vi "LevMar - TestSuite.vi"() -> ()   [LabVIEW 2009]
uses:
  <vilib>/Analysis/NI_AALBase.lvlib
panel:
  out "Reduced Chi2":dbl(graph)=0.8280414251118929
  out "Graphe XY":T1(graph)=[{"Ramp Pattern"=[-1.0, -0.9797979797979798, -0.9595959595959596, -0.9393939393939393, -0.9191919191919191, -0.8989898989898989, -0.8787878787878787, -0.8585858585858585, -0.8383838383838382, -0.818181818181818, -0.7979797979797978, -0.7777777777777776, -0.7575757575757573, -0.7373737373737371, -0.7171717171717169, -0.6969696969696967, -0.6767676767676765, -0.6565656565656562, -0.636363636363636, -0.6161616161616158, -0.5959595959595956, -0.5757575757575754, -0.5555555555555551, -0.5353535353535349, -0.5151515151515147, -0.4949494949494945, -0.47474747474747425, -0.45454545454545403, -0.4343434343434338, -0.4141414141414136, -0.39393939393939337, -0.37373737373737315, -0.3535353535353529, -0.3333333333333327, -0.3131313131313125, -0.29292929292929226, -0.27272727272727204, -0.2525252525252518, -0.23232323232323163, -0.21212121212121143, -0.19191919191919124, -0.17171717171717105, -0.15151515151515085, -0.13131313131313066, -0.11111111111111045, -0.09090909090909025, -0.07070707070707004, -0.05050505050504983, -0.030303030303029627, -0.010101010101009424, 0.01010101010101078, 0.030303030303030984, 0.05050505050505119, 0.0707070707070714, 0.0909090909090916, 0.11111111111111181, 0.13131313131313202, 0.1515151515151522, 0.1717171717171724, 0.1919191919191926, 0.2121212121212128, 0.232323232323233, 0.2525252525252532, 0.27272727272727343, 0.29292929292929365, 0.31313131313131387, 0.3333333333333341, 0.3535353535353543, 0.37373737373737453, 0.39393939393939476, 0.414141414141415, 0.4343434343434352, 0.4545454545454554, 0.47474747474747564, 0.49494949494949586, 0.515151515151516, 0.5353535353535362, 0.5555555555555565, 0.5757575757575767, 0.5959595959595969, 0.6161616161616171, 0.6363636363636374, 0.6565656565656576, 0.6767676767676778, 0.696969696969698, 0.7171717171717182, 0.7373737373737385, 0.7575757575757587, 0.7777777777777789, 0.7979797979797991, 0.8181818181818193, 0.8383838383838396, 0.8585858585858598, 0.87878787878788, 0.8989898989899002, 0.9191919191919204, 0.9393939393939407, 0.9595959595959609, 0.9797979797979811, 1.0000000000000013], "Best Fit"=[-0.0016898079029579738, -0.010518321765782213, -0.01737091840455096, -0.022296729825936557, -0.025344888036609614, -0.026564525043242138, -0.026004772852505242, -0.023714763471070988, -0.019743628905610155, -0.01414050116279486, -0.006954512249295941, 0.0017652058282146, 0.011969521063065702, 0.023609301448585474, 0.03663541497810291, 0.05099872964494598, 0.06665011344244379, 0.08354043436392442, 0.10162056040271661, 0.12084135955214889, 0.14115369980554973, 0.16250844915624768, 0.18485647559757126, 0.20814864712284895, 0.2323358317254094, 0.257368897398581, 0.2831987121356923, 0.3097761439300718, 0.3370520607750481, 0.36497733066394983, 0.3935028215901053, 0.4225794015468432, 0.452157938527492, 0.4821893005253801, 0.5126243555338362, 0.5434139715461888, 0.5745090165557664, 0.6058603585558975, 0.6374188655399105, 0.6691354055011342, 0.7009608464328968, 0.7328460563285272, 0.7647419031813537, 0.7965992549847049, 0.8283689797319093, 0.8600019454162954, 0.8914490200311918, 0.9226610715699269, 0.9535889680258294, 0.9841835773922277, 1.0143957676624504, 1.0441764068298258, 1.0734763628876829, 1.1022465038293496, 1.130437697648155, 1.1580008123374275, 1.1848867158904952, 1.211046276300687, 1.2364303615613315, 1.260989839665757, 1.2846755786072923, 1.3074384463792654, 1.3292293109750055, 1.3499990403878406, 1.3696985026110995, 1.3882785656381107, 1.4056900974622026, 1.421883966076704, 1.436811039474943, 1.4504221856502484, 1.4626682725959488, 1.4735001683053726, 1.4828687407718482, 1.4907248579887042, 1.4970193879492693, 1.5017031986468719, 1.5047271580748405, 1.5060421342265038, 1.50559899509519, 1.5033486086742278, 1.499241842956946, 1.4932295659366728, 1.4852626456067366, 1.4752919499604662, 1.4632683469911902, 1.4491427046922367, 1.4328658910569347, 1.4143887740786125, 1.3936622217505985, 1.3706371020662216, 1.34526428301881, 1.317494632601692, 1.287279018808197, 1.254568309631653, 1.219313373065388, 1.1814650771027315, 1.1409742897370114, 1.0977918789615562, 1.051868712769695, 1.0031556591547555]}, {"Ramp Pattern"=[-1.0, -0.9797979797979798, -0.9595959595959596, -0.9393939393939393, -0.9191919191919191, -0.8989898989898989, -0.8787878787878787, -0.8585858585858585, -0.8383838383838382, -0.818181818181818, -0.7979797979797978, -0.7777777777777776, -0.7575757575757573, -0.7373737373737371, -0.7171717171717169, -0.6969696969696967, -0.6767676767676765, -0.6565656565656562, -0.636363636363636, -0.6161616161616158, -0.5959595959595956, -0.5757575757575754, -0.5555555555555551, -0.5353535353535349, -0.5151515151515147, -0.4949494949494945, -0.47474747474747425, -0.45454545454545403, -0.4343434343434338, -0.4141414141414136, -0.39393939393939337, -0.37373737373737315, -0.3535353535353529, -0.3333333333333327, -0.3131313131313125, -0.29292929292929226, -0.27272727272727204, -0.2525252525252518, -0.23232323232323163, -0.21212121212121143, -0.19191919191919124, -0.17171717171717105, -0.15151515151515085, -0.13131313131313066, -0.11111111111111045, -0.09090909090909025, -0.07070707070707004, -0.05050505050504983, -0.030303030303029627, -0.010101010101009424, 0.01010101010101078, 0.030303030303030984, 0.05050505050505119, 0.0707070707070714, 0.0909090909090916, 0.11111111111111181, 0.13131313131313202, 0.1515151515151522, 0.1717171717171724, 0.1919191919191926, 0.2121212121212128, 0.232323232323233, 0.2525252525252532, 0.27272727272727343, 0.29292929292929365, 0.31313131313131387, 0.3333333333333341, 0.3535353535353543, 0.37373737373737453, 0.39393939393939476, 0.414141414141415, 0.4343434343434352, 0.4545454545454554, 0.47474747474747564, 0.49494949494949586, 0.515151515151516, 0.5353535353535362, 0.5555555555555565, 0.5757575757575767, 0.5959595959595969, 0.6161616161616171, 0.6363636363636374, 0.6565656565656576, 0.6767676767676778, 0.696969696969698, 0.7171717171717182, 0.7373737373737385, 0.7575757575757587, 0.7777777777777789, 0.7979797979797991, 0.8181818181818193, 0.8383838383838396, 0.8585858585858598, 0.87878787878788, 0.8989898989899002, 0.9191919191919204, 0.9393939393939407, 0.9595959595959609, 0.9797979797979811, 1.0000000000000013], "Best Fit"=[0.0068763694567000105, -0.013757383340708685, -0.0272231962940259, -0.021606159820455873, -0.029952272522872393, -0.02794214384950997, -0.041467239064541625, -0.021168592799294707, -0.02474381389419588, 0.00267259751288184, -0.0010875078317083104, 0.006935196863699051, 0.02371014280289723, 0.024350215775652204, 0.035589174010403776, 0.06445808144428938, 0.07683458790373367, 0.08183637710296356, 0.09127531613198694, 0.12416245979065038, 0.1383160631505338, 0.15870717638953083, 0.18896831456394578, 0.19214243850283919, 0.2459083674187535, 0.2547635484506904, 0.2705573482370152, 0.3140520910654134, 0.34446844589872927, 0.3503785326623043, 0.3774173461312958, 0.41026332139838784, 0.4573052751472374, 0.4806701569394728, 0.49319035392745986, 0.5473355214834735, 0.5814913095186334, 0.6003332277431696, 0.6359363831011836, 0.6847120296522752, 0.6979898441718131, 0.7318336707796799, 0.7678382522048454, 0.806270615423049, 0.8227181691173335, 0.8648107494305103, 0.885698597958113, 0.9444874055653282, 0.9678084783900404, 0.9870660398026526, 1.0117064267265494, 1.02885879678619, 1.0776699526365756, 1.103032050385832, 1.1240294227010545, 1.1579427056971643, 1.198048582057967, 1.2004426344631474, 1.239306308869129, 1.2679423130993166, 1.2862664199719294, 1.3089566783906899, 1.3296856943335784, 1.3477340839541145, 1.3501324109053527, 1.4024117914777718, 1.3990612113567793, 1.4177994589161165, 1.4536408827705687, 1.4428389277741696, 1.459603383882423, 1.4790749393406786, 1.4688628194274158, 1.4779910036411437, 1.4886019053135138, 1.5192068140825437, 1.5056057062591697, 1.5112645805524276, 1.5059178390597947, 1.5131001873938164, 1.5000642610260897, 1.5006317922343897, 1.49826796404352, 1.4847408656101546, 1.4584376620416672, 1.4451782789969199, 1.4212354477953029, 1.3992929656483506, 1.3888595982023753, 1.358099138788165, 1.3392365798120078, 1.3158770982609125, 1.2900307263125528, 1.2521637211322305, 1.2347895389871848, 1.1717961456379768, 1.1433511019909486, 1.1082589909107459, 1.0540896400505515, 1.0037091247691126]}]
  in  "standard deviation":dbl=0.009999999999999997 caption="écart-type" format="%.6f"
  out "Best Fit Coefficients":dbl[](array[numeric])=[0.9993405456647769, 1.4956047531397814, -0.49860762003887654, -0.993182019610923] caption="Coefficients d'ajustement optimaux" format="%_6f"
  in  "A":dbl[](array[numeric])=[1.0, 1.5, -0.5, -1.0]
  in  "samples":i32=100 caption="échantillons"
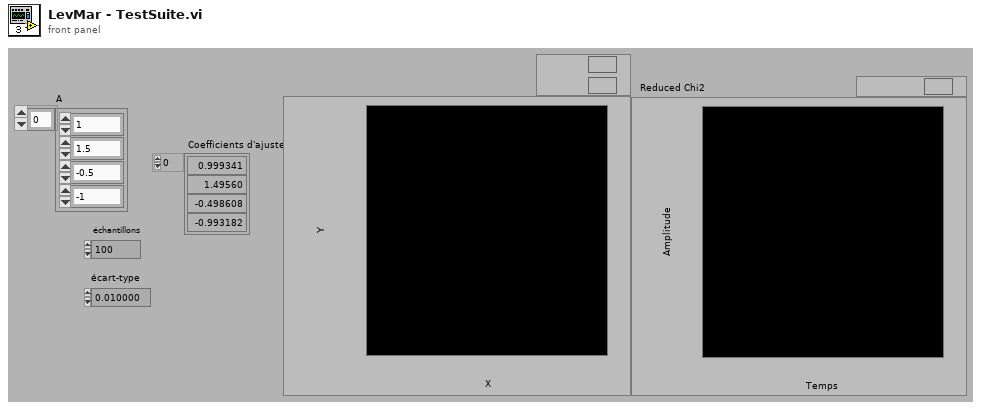
[diagram p1: front panel]
types:
  T1 = cluster{"Ramp Pattern":dbl[], "Best Fit":dbl[]}[]
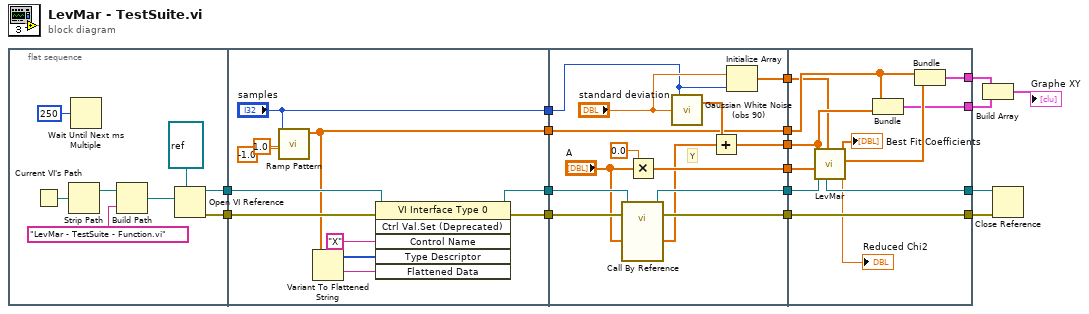
[diagram p0: block diagram]
diagram:
  n1 = flat-sequence {
    tunnel: [w20] -> w17
    tunnel: [w19] -> w16
    tunnel: w16 -> [w34]
    tunnel: w17 -> [w35]
    tunnel: [w35] -> w15
    tunnel: [w33] -> w14
    tunnel: ["samples"] -> w7
    tunnel: [w26] -> w6
    tunnel: w15 -> [w48]
    tunnel: w14 -> [w47]
    tunnel: [w48] -> w13
    tunnel: [w46] -> w12
    tunnel: [w44] -> w11
    tunnel: [w41] -> w10
    tunnel: w7 -> [w37]
    tunnel: w6 -> [w39]
    tunnel: [w39] -> w5
    tunnel: [w36] -> w1
    tunnel: [w57] -> w8
    tunnel: [w60] -> w9
    tunnel: w13 -> [w60]
    tunnel: w12 -> [w58]
    tunnel: w11 -> [w59]
    tunnel: w10 -> [w56]
    tunnel: w5 -> [w55]
    tunnel: [w53] -> w2
    tunnel: [w52] -> w3
    tunnel: w1 -> [w50]
    frame #0 {
      n2 = Current VI's Path() -> (path=w25:path)
      n3 = Strip Path(path=w25) -> (stripped path=w24:path)  [unwired: 1 out]
      n4 = Wait Until Next ms Multiple(millisecond multiple=u32 250 ("n millisecondes")) -> ()  [unwired: 1 out]
      n5 = Build Path(base path=w24, name or relative path="LevMar - TestSuite - Function.vi" ("nom ou chemin relatif")) -> (appended path=w22:path)
      n6 = Open VI Reference(type specifier VI Refnum (for type only)=refnum<vi> refnum ("Refnum de VI spécificateur de type (pour type seulement)"), vi path=w22) -> (vi reference=w19:refnum<vi>, error out=w20:errorcluster)  [unwired: 4 in]
    }
    frame #1 {
      n7 = call <vilib>:"Ramp Pattern.vi"("start"=-1.0, "end"=1.0, "samples"="samples") -> ("Ramp Pattern"=w26:dbl[])  [unwired: 7 in, 1 out]
      n8 = Variant To Flattened String(Variant=w26) -> (data string=w30:string, 1:w31:i16[])
      n9 = invoke class="VI Interface Type 0" method="Ctrl Val.Set (Deprecated)"(reference=w34, error in=w35, "Control Name"="X" ("Nom de la commande"), "Type Descriptor"=w31, "Flattened Data"=w30) -> (reference out=w33:refnum<vi>)  [unwired: 1 in, 5 out]
    }
    frame #2 {
      # "Y"
      n10 = call-by-ref "?"(reference=w47, error in=w48, "A"="A") -> (reference out=w46:refnum<vi>, "F"=w42:dbl[])  [unwired: 1 out]
      n11 = Multiply(x=0.0, y="A") -> (x*y=w44:dbl[])
      n12 = call <vilib>:"Gaussian White Noise (obs 90).vi"("standard deviation"="standard deviation", "samples"=w37) -> ("Gaussian noise pattern"=w40:dbl[])  [unwired: 1 in, 1 out]
      n13 = Add(x=w40, y=w42) -> (x+y=w41:dbl[])
      n14 = Initialize Array("standard deviation", w37) -> (w36:dbl[])
    }
    frame #3 {
      n15 = call "LevMar.vi"("Standard Deviation"=w50, "Initial Guess Coefficients"=w59, "Y"=w56, "Target function in"=w58) -> ("mse"=→"Reduced Chi2":dbl, "Best Fit"=w54:dbl[], "Best Fit Coefficients"=→"Best Fit Coefficients":dbl[], "Target function out"=w57:refnum<vi>)  [unwired: 1 in, 2 out]
      n16 = Bundle("Ramp Pattern"=w55, w56) -> (w53:cluster{"Ramp Pattern":dbl[], dbl[]})  [unwired: 1 in]
      n17 = Bundle("Ramp Pattern"=w55, "Best Fit"=w54) -> (w52:cluster{"Ramp Pattern":dbl[], "Best Fit":dbl[]})  [unwired: 1 in]
    }
  }
  n18 = Build Array(w3, w2) -> (→"Graphe XY":T1)
  n19 = Close Reference(reference=w8, error in (no error)=w9) -> ()  [unwired: 1 out]
